vi "Tank.vi"() -> ()   [LabVIEW 2018]
panel:
  in  "stop":bool
  out "Numeric 2":i16
  in  "Numeric":u64
  in  "Débit":i16(slide) min=0 max=10 scale=0.0..10.0
  in  "Consigne":i16(slide) scale=0.0..1000.0
  in  "Tank":i16(slide) scale=0.0..1000.0
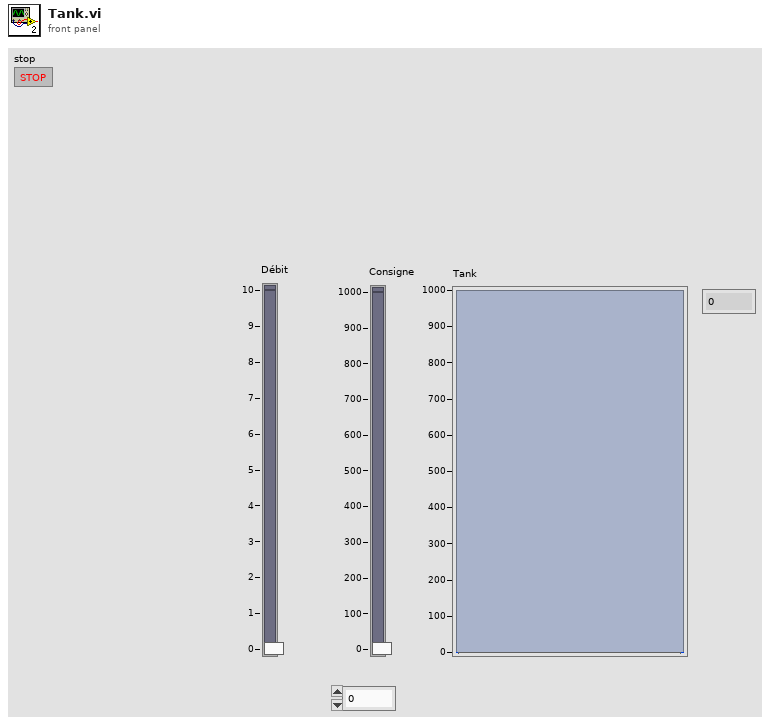
[diagram p1: front panel]
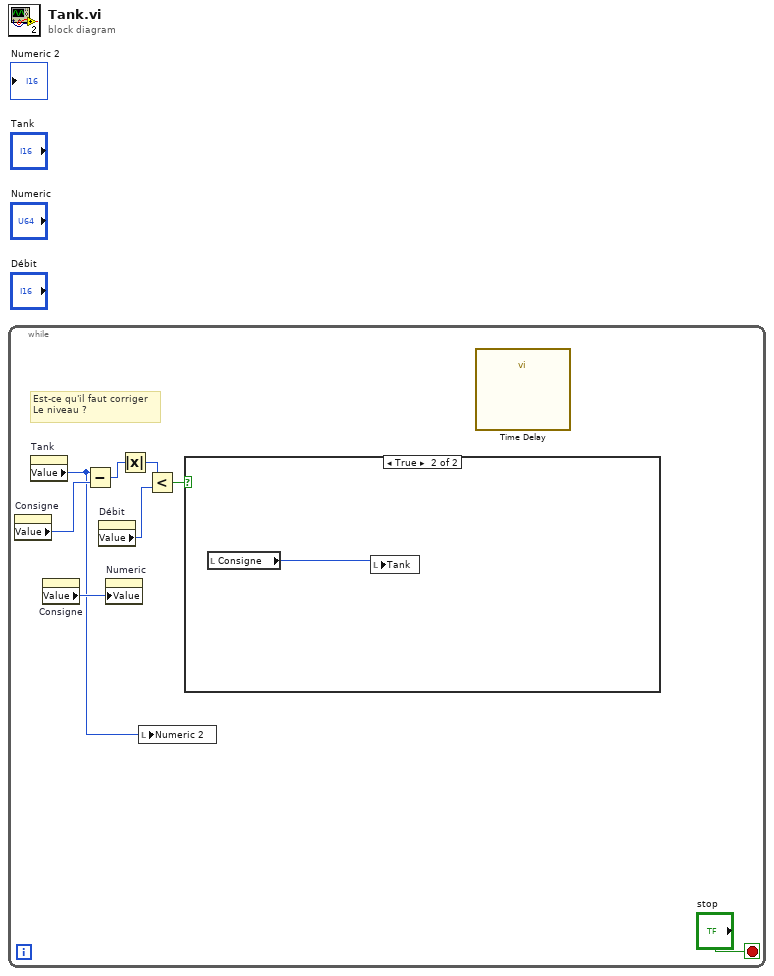
[diagram p0: block diagram]
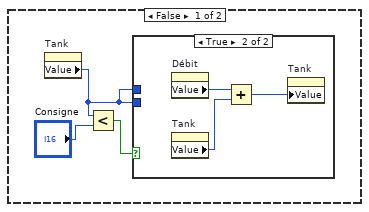
[diagram p2: hidden frame]
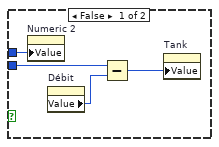
[diagram p3: hidden frame]
diagram:
  n1 = while {
    stop <- "stop" stop-if-true
    # "Est-ce qu'il faut corriger\nLe niveau ?"
    n2 = property on="Consigne" class="Slide (strict)"() -> ("Value"=w5:i16)  [unwired: 2 in, 2 out]
    n3 = property on="Tank" class="Slide (strict)"() -> ("Value"=w1:i16)  [unwired: 2 in, 2 out]
    n4 = property on="Consigne" class="Slide (strict)"() -> ("Value"=w7:i16)  [unwired: 2 in, 2 out]
    n5 = Subtract(x=w1, y=w5) -> (x-y=w4:i16)
    n6 = property on="Débit" class="Slide (strict)"() -> ("Value"=w6:i16)  [unwired: 2 in, 2 out]
    n7 = property on="Numeric" class="DigNum (strict)"("Value"=w7) -> ()  [unwired: 2 in, 2 out]
    n8 = Absolute Value(x=w4) -> (abs(x)=w3:i16)
    n9 = local write "Numeric 2"(w1) -> ()
    n10 = Less?(x=w3, y=w6) -> (x < y?=w2:bool)
    n11 = case shown="True" w2 {
      frame False {
        n12 = property on="Tank" class="Slide (strict)"() -> ("Value"=w10:i16)  [unwired: 2 in, 2 out]
        n13 = Less?(x=w10, y="Consigne") -> (x < y?=w9:bool)
        n14 = case shown="True" w9 {
          tunnel: w10 -> [w13 _]
          tunnel: w10 -> [w12 _]
          frame False {
            n15 = property on="Numeric 2" class="DigNum (strict)"("Value"=w12) -> ()  [unwired: 2 in, 2 out]
            n16 = property on="Débit" class="Slide (strict)"() -> ("Value"=w15:i16)  [unwired: 2 in, 2 out]
            n17 = Subtract(x=w13, y=w15) -> (x-y=w14:i16)
            n18 = property on="Tank" class="Slide (strict)"("Value"=w14) -> ()  [unwired: 2 in, 2 out]
          }
          frame True {
            n19 = property on="Débit" class="Slide (strict)"() -> ("Value"=w17:i16)  [unwired: 2 in, 2 out]
            n20 = property on="Tank" class="Slide (strict)"() -> ("Value"=w16:i16)  [unwired: 2 in, 2 out]
            n21 = Add(x=w17, y=w16) -> (x+y=w18:u32)
            n22 = property on="Tank" class="Slide (strict)"("Value"=w18) -> ()  [unwired: 2 in, 2 out]
          }
        }
      }
      frame True {
        n23 = local read "Consigne"() -> (w19:i16)
        n24 = local write "Tank"(w19) -> ()
      }
    }
    n25 = call "Time Delay"() -> ()  [unwired: 11 in, 1 out]
  }
